vi "Quit GNU Octave.vi"(8 "error in":errorcluster, 11 "GOLPI ref. in":T1={"pipe handle"={"lv_proc.dll file path"=path "", "process instance handle"=[]}, "fast read timeout [ms]"=500, "fast read settle time [ms]"=10, "fast read to multiple [ms]"=1, "max elements per input line"=100, "slow read timeout [ms]"=5000, "stdin double format specifier"="%_16e", "max elements per stdout output column"=100}) -> (0 "error out":errorcluster, 2 "exit code":i32)   [LabVIEW 2013, in "GOLPI library.lvlib"]
doc: "Quits GNU Octave by any means. First sends command 'exit', if not sucessfull closes or kills the GNU Octave process."
uses:
  GOLPI library.lvlib
  Private/Type Definitions/GOLPI reference Type Def.ctl
  LV Process source distribution/Pipe Handle.ctl
  LV Process source distribution/LV Process library.lvlib
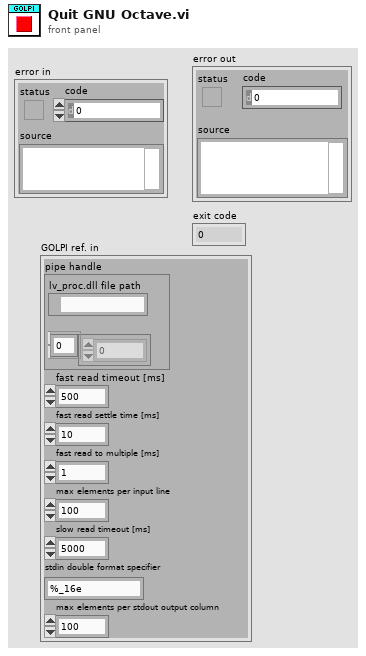
[diagram p1: front panel]
types:
  T1 = typedef "GOLPI library.lvlib/GOLPI reference Type Def.ctl" = cluster{"pipe handle":T2, "fast read timeout [ms]":u32, "fast read settle time [ms]":u32, "fast read to multiple [ms]":u32, "max elements per input line":u32, "slow read timeout [ms]":u32, "stdin double format specifier":string, "max elements per stdout output column":u32}
  T2 = typedef "LV Process library.lvlib/Pipe Handle.ctl" = cluster{"lv_proc.dll file path":path, "process instance handle":u32[]}
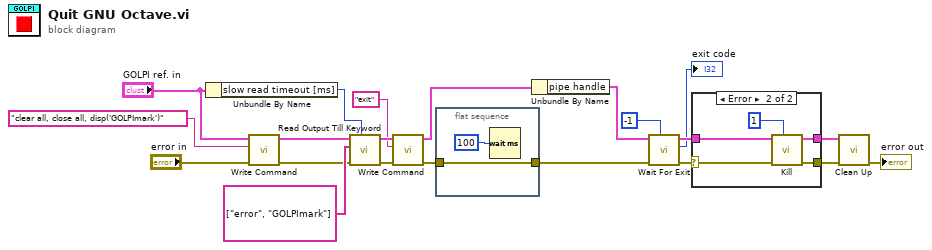
[diagram p0: block diagram]
diagram:
  n1 = Unbundle By Name("GOLPI ref. in") -> ("slow read timeout [ms]"=w1:u32)
  n2 = call "Write Command.vi"("error in"="error in", "command"="clear all, close all, disp('GOLPImark')" ("write buffer"), "GOLPI ref. in"="GOLPI ref. in") -> ("error out"=w10:errorcluster, "GOLPI ref. out"=w9:T1)  [unwired: 7 in]
  n3 = call "Read Output Till Keyword.vi"("timeout [ms]"=w1, "error in"=w10, "keywords"=string[] ["error", "GOLPImark"], "GOLPI ref. in"=w9) -> ("error out"=w7:errorcluster, "GOLPI ref. out"=w8:T1)  [unwired: 4 in, 2 out]
  n4 = call "Write Command.vi"("error in"=w7, "command"="exit", "GOLPI ref. in"=w8) -> ("error out"=w3:errorcluster, "GOLPI ref. out"=w5:T1)  [unwired: 7 in]
  n5 = flat-sequence {
    tunnel: [w22] -> w14
    tunnel: w3 -> [w22]
    frame #0 {
      n6 = Wait (ms)(milliseconds to wait=u32 100) -> ()  [unwired: 1 out]
    }
  }
  n7 = Unbundle By Name(w5) -> ("pipe handle"=w4:T2)
  n8 = call "Wait For Exit.vi"("timeout [ms]"=-1, "error in"=w14, "pipe in"=w4) -> ("error out"=w19:errorcluster, "exit code"=→"exit code":i32, "pipe out"=w18:T2)  [unwired: 6 in]
  n9 = case shown="Error" w19 {
    selector: w19 -> [w24 w29]
    tunnel: w18 -> [w25 w28]
    tunnel: [w24 w30] -> w20
    tunnel: [w25 w27] -> w16
    frame No Error {
    }
    frame Error {
      n10 = call "Kill.vi"("timeout [ms]"=1, "error in"=w29, "pipe in"=w28) -> ("error out"=w30:errorcluster, "pipe out"=w27:T2)  [unwired: 7 in]
    }
  }
  n11 = call "Clean Up.vi"("error in"=w20, "pipe in"=w16) -> ("error out"=→"error out":errorcluster)  [unwired: 9 in]
